vi "prime composite odd even.vi"() -> ()   [LabVIEW 2018]
panel:
  out "Composite number":i32[](array[numeric])
  out "Prime Numbers":i32[](array[numeric])
  out "odd":i32[](array[numeric])
  out "even":i32[](array[numeric])
  in  "Numeric":dbl
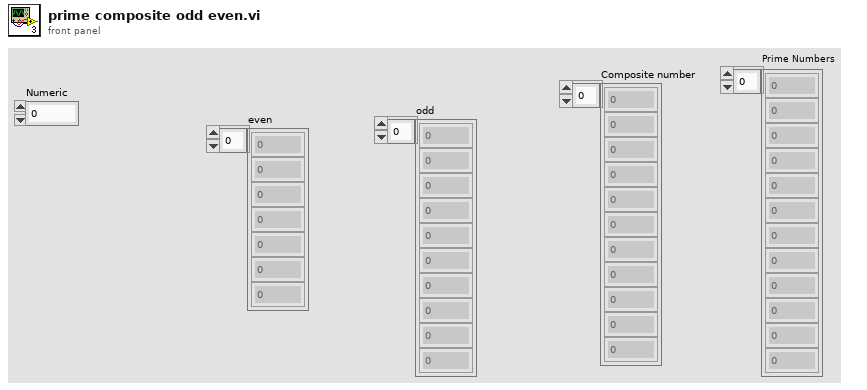
[diagram p1: front panel]
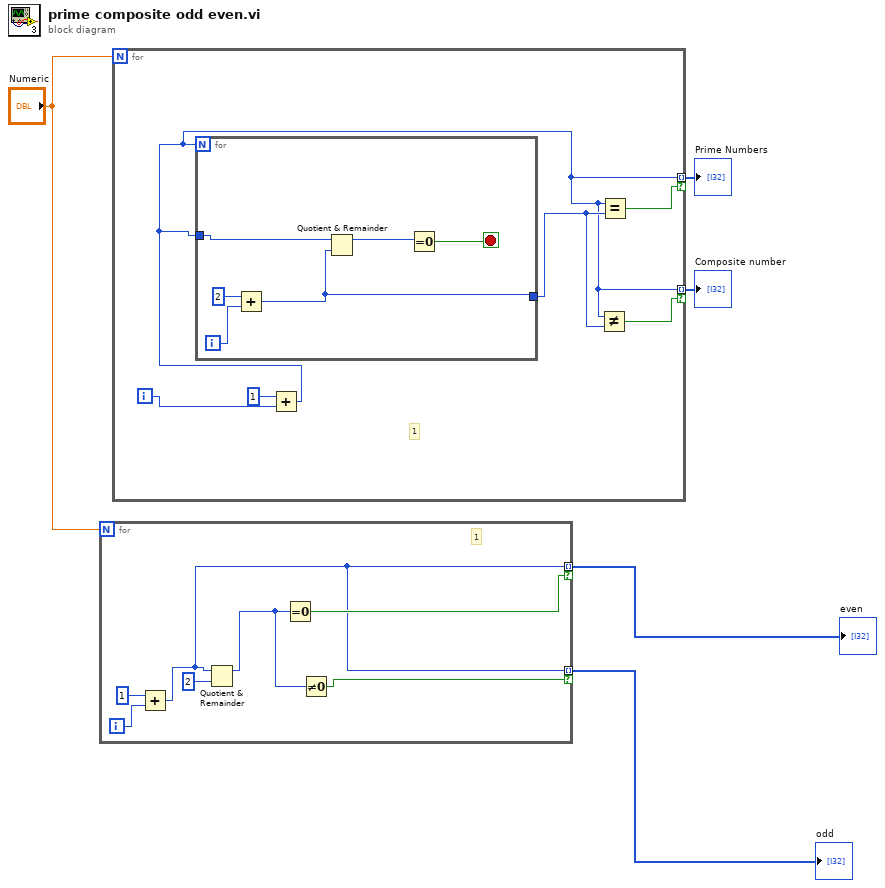
[diagram p0: block diagram]
diagram:
  n1 = for {
    N: "Numeric" -> [_]
    tunnel: [w6] -> w5 mode=indexing if=w9
    tunnel: [w6] -> w4 mode=indexing if=w7
    i -> [w11]
    # "1"
    n2 = Add(x=1, y=w11) -> (x+y=w6:i32)
    n3 = Quotient & Remainder(x=w6, y=2) -> (x-y*floor(x/y)=w8:i32)  [unwired: 1 out]
    n4 = Equal To 0?(x=w8) -> (x = 0?=w9:bool)
    n5 = Not Equal To 0?(x=w8) -> (x != 0?=w7:bool)
  }
  "even" <- w5
  "odd" <- w4
  n6 = for {
    N: "Numeric" -> [_]
    tunnel: [w13] -> w3 mode=indexing if=w17
    tunnel: [w13] -> w2 mode=indexing if=w16
    i -> [w15]
    # "1"
    n7 = Add(x=1, y=w15) -> (x+y=w13:i32)
    n8 = for {
      N: w13 -> [_]
      tunnel: w13 -> [w20]
      tunnel: [w19] -> w18
      i -> [w22]
      stop <- w24 stop-if-true
      n9 = Add(x=2, y=w22) -> (x+y=w19:i32)
      n10 = Quotient & Remainder(x=w20, y=w19) -> (x-y*floor(x/y)=w23:i32)  [unwired: 1 out]
      n11 = Equal To 0?(x=w23) -> (x = 0?=w24:bool)
    }
    n12 = Not Equal?(x=w13, y=w18) -> (x != y?=w16:bool)
    n13 = Equal?(x=w13, y=w18) -> (x = y?=w17:bool)
  }
  "Prime Numbers" <- w3
  "Composite number" <- w2
